vi "Name Value Check New.vi"(0 "Tags":string[](array[string]), 5 "Sorted Tags":string[](array[string]), 7 "First Letters":string[](array[string]), 9 "Letter Indicies":i32[](array[numeric])) -> (8 "New Tags":string[](array[string]), 15 "New Tags Bool":bool)   [LabVIEW 2020]
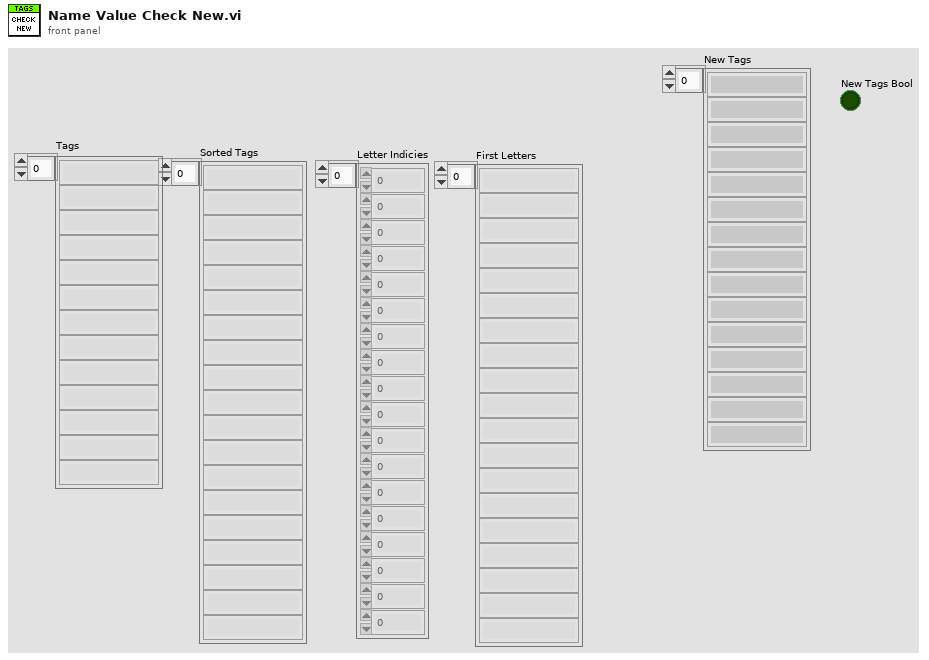
[diagram p1: front panel]
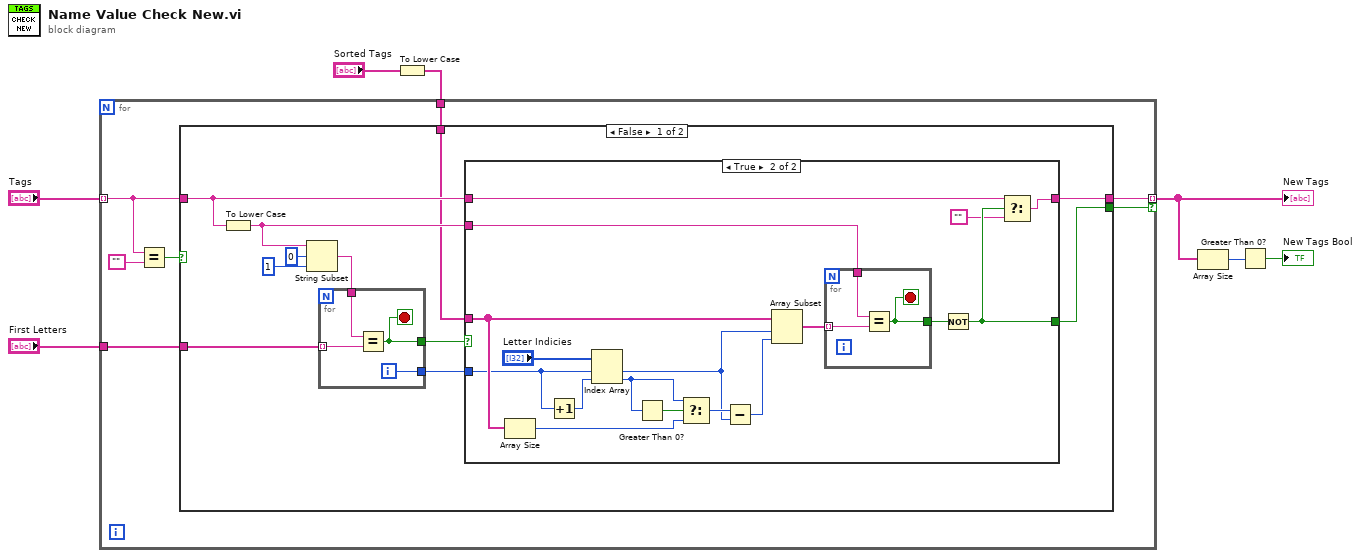
[diagram p0: block diagram]
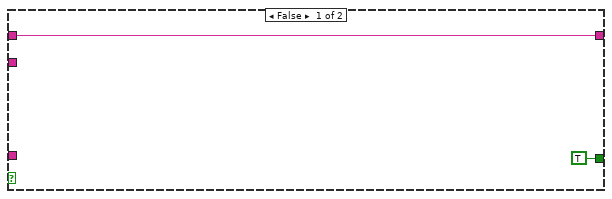
[diagram p2: hidden frame]
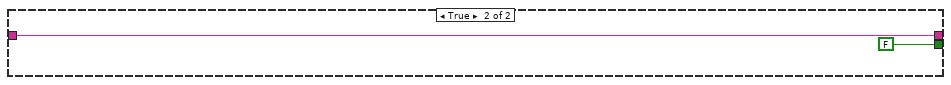
[diagram p3: hidden frame]
diagram:
  n1 = To Lower Case(string="Sorted Tags") -> (all lower case string=w5:string[])
  n2 = for {
    tunnel: "Tags" -> [w10] mode=indexing
    tunnel: [w14] -> w4 mode=indexing if=w13
    tunnel: w5 -> [w12]
    tunnel: "First Letters" -> [w11]
    n3 = Equal?(x=w10, y="") -> (x = y?=w8:bool)
    n4 = case shown="False" w8 {
      tunnel: w10 -> [w19 w53]
      tunnel: [w18 w53] -> w14
      tunnel: [w17 FALSE] -> w13
      tunnel: w12 -> [w16 _]
      tunnel: w11 -> [w15 _]
      frame False {
        n5 = To Lower Case(string=w19) -> (all lower case string=w20:string)
        n6 = String Subset(string=w20, offset (0)=0, length (rest)=1 ("length (rest)")) -> (substring=w23:string)
        n7 = for {
          tunnel: w15 -> [w51] mode=indexing
          tunnel: w23 -> [w50]
          tunnel: [w49] -> w22
          tunnel: [w48] -> w21
          i -> [w48]
          stop <- w49 stop-if-true
          n8 = Equal?(x=w50, y=w51) -> (x = y?=w49:bool)
        }
        n9 = case shown="True" w22 {
          tunnel: w16 -> [_ w38]
          tunnel: w21 -> [_ w35]
          tunnel: w19 -> [w27 w30]
          tunnel: [w27 w29] -> w18
          tunnel: w20 -> [_ w33]
          tunnel: [TRUE w31] -> w17
          frame False {
          }
          frame True {
            n10 = Array Size(array=w38) -> (size(s)=w40:i32)
            n11 = Increment(x=w35) -> (x+1=w43:i32)
            n12 = Index Array(array="Letter Indicies", index #1=w35, index #2=w43) -> (element #1=w36:i32, element #2=w41:i32)
            n13 = Greater Than 0?(x=w41) -> (x > 0?=w42:bool)
            n14 = Select(t=w41, s=w42, f=w40) -> (s? t:f=w39:i32)
            n15 = Subtract(x=w39, y=w36) -> (x-y=w37:i32)
            n16 = Array Subset(array=w38, index=w36, length=w37) -> (w34:string[])
            n17 = for {
              tunnel: w34 -> [w47] mode=indexing
              tunnel: w33 -> [w46]
              tunnel: [w45] -> w32
              stop <- w45 stop-if-true
              n18 = Equal?(x=w46, y=w47) -> (x = y?=w45:bool)
            }
            n19 = Not(x=w32) -> (.not. x?=w31:bool)
            n20 = Select(t=w30, s=w31, f="") -> (s? t:f=w29:string)
          }
        }
      }
      frame True {
      }
    }
  }
  "New Tags" <- w4
  n21 = Array Size(array=w4) -> (size(s)=w3:i32)
  n22 = Greater Than 0?(x=w3) -> (x > 0?=→"New Tags Bool":bool)
